vi "Main.vi"   [LabVIEW 2023]
uses:
  Control 1.ctl
types:
  T1 = typedef "Control 1.ctl" = enum16{"int", "read", "write", "Kundeneingabe", "Betonauswahl", "Bezahlprozess", " Rechnung", "Zutaten hinzufügen", "Stop"}
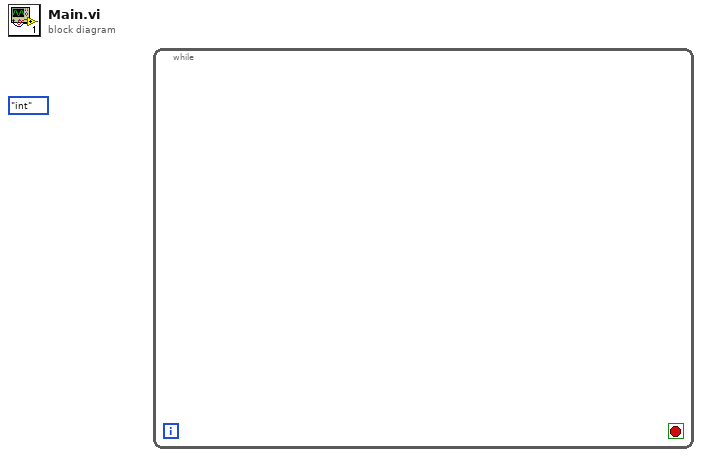
[diagram p0: block diagram]
diagram:
  (unwired) Control_1."int"
  n1 = while {
    stop <- _ stop-if-true
  }
